vi "Test TestStand Manager_DQMH API.vi"   [LabVIEW 2015]
doc: "TestStand Manager_DQMH API Tester.\n\nThis VI would normally be used to test the API for the Module.\n\nHowever, the TestStand Manager_DQMH has a modified Start Module.vi that takes the Sequence Context reference directly from the executing TestStand sequence. \n\nTo be able to replicate this in a LabVIEW API tester, we would need to add code to invoke the TestStand engine and then open and run a dummy sequence to then obtain its sequence.\nThis is different than how we are using the module.\n\nThe purpose of the TestStand Manager_DQMH Module is to check if the TestStand sequence is terminated. If so, it sends the request to stop all Thermal Chamber DQMH modules. This Module is only used when running the TestStand Examples.\n____\nDelacor QMH Thermal Chamber Examples 4.0.0.21\nCopyright (c) 2018, Delacor"
uses:
  TestStand Manager_DQMH.lvlib
panel:
  # "This VI would normally be used to test the API for the Module.\n\nHowever, the TestStand Manager_DQMH has a modified Start Module.vi that takes the Sequence Context reference directly from the executing TestStand sequence. \n\nTo be able to replicate this in a LabVIEW API tester, we would need to add code to invoke the TestStand engine and then open and run a dummy sequence to then obtain its sequence.\nThis is different than how we are using the module.\n\nThe purpose of the TestStand Manager_DQMH Module is to check if the TestStand sequence is terminated. If so, it sends the request to stop all Thermal Chamber DQMH modules. This Module is only used when running the TestStand Examples."
types:
  T1 = typedef "TestStand Manager_DQMH.lvlib/Broadcast Events--cluster.ctl" = cluster{"Module Did Init":refnum<user-event>, "Status Updated":refnum<user-event>, "Error Reported":refnum<user-event>, "Module Did Stop":refnum<user-event>, "Update Module Execution Status":refnum<user-event>}
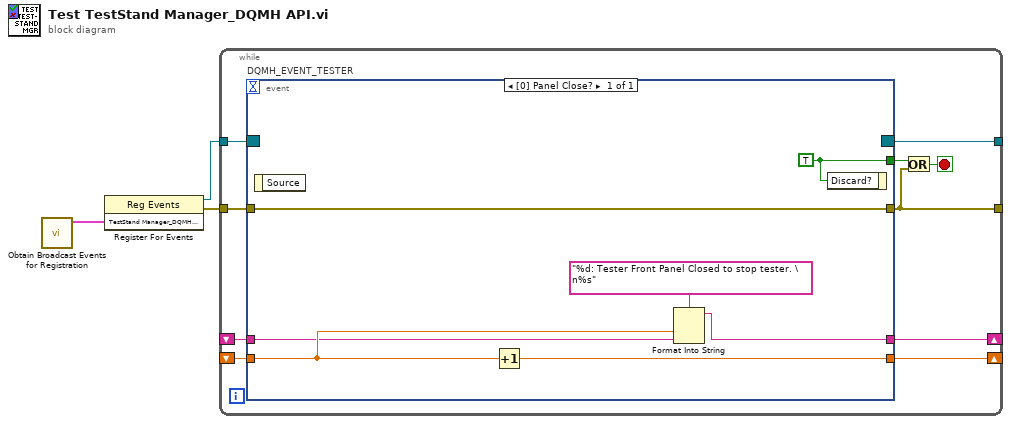
[diagram p0: block diagram]
diagram:
  n1 = call "Obtain Broadcast Events for Registration.vi"() -> ("TestStand Manager_DQMH Broadcast Events"=w1:T1)  [unwired: 9 in, 2 out]
  n2 = register-events(w1) -> (reference out=w2:refnum<event-registration>, error out=w3:errorcluster)  [unwired: 2 in]
  n3 = while {
    tunnel: w2 -> [w13]
    tunnel: [w6] -> _
    shift-right: [w8] -> _
    shift-left: _ -> [w10]
    shift-right: [w9] -> _
    shift-left: _ -> [w11]
    tunnel: w3 -> [w5]
    tunnel: [w4] -> _
    stop <- w7 stop-if-true
    n4 = event "DQMH_EVENT_TESTER" shown="[0] Panel Close?" {
      selector: w13 -> [_]
      dyn-events: [_] -> w4
      timeout: _ -> [_]
      tunnel: [w20] -> w12
      tunnel: [w19] -> w6
      tunnel: w11 -> [w17]
      tunnel: w10 -> [w15]
      tunnel: [w14] -> w8
      tunnel: [w16] -> w9
      tunnel: w5 -> [w19]
      event Panel Close? {
        w20 = TRUE ("Discard?")
        n5 = event-data() -> ()  [unwired: 1 in, 1 out]
        n6 = Increment(x=w17) -> (x+1=w16:dbl)
        n7 = Format Into String(format string="%d: Tester Front Panel Closed to stop tester. \n%s", w17, w15) -> (resulting string=w14:string)  [unwired: 2 in, 1 out]
        n8 = event-data("Discard?"=w20) -> ()  [unwired: 1 in, 1 out]
      }
    }
    n9 = Or(x=w12, y=w6) -> (x .or. y?=w7:bool)
  }
